vi "Main.vi"(11 "Module Admin":refnum<class "Delacor_lib_QMH_Module Admin.lvclass">) -> ()   [LabVIEW 2019, in "ContextHelp.lvlib"]
doc: "This template is based off of the Queued Message Handler design pattern and the Queued Message Handler project template that ships with LabVIEW.\n\nThe main difference is that the queue is private to this module and communication between modules is performed via Broadcast and Request events.\n\nRequest events are wrapped in public API methods and are handled in the Event Handling Loop (EHL) of this VI. Any module can register for Broadcast events sent by this module. The EHL generates messages based on user interface actions.\n\nThe Message Handling Loop (MHL) processes messages generated by the EHL, or by other messages. The messages are string values, so new messages can be added easily to the Message Cases case structure in the MHL. Each message cluster can also provide an optional value for Message Data, which is a variant that can be converted to whatever message-specific data is required.\n_____\nBased on DQMH Project Template 6.1.0.94.\n____\nPantherLAB Templates 1.0.0.5\nCopyright (c) 2022, PantherLAB\n\n<b>Note:</b> This VI was modified by the <b>Validate DQMH Module</b> tool to add a 'Panel Hidden' status updated broadcast to the Panel Close? event when External Launch = TRUE.\n\n<b>Note:</b> This VI was modified by the <b>Validate DQMH Module</b> tool to add a call to the Error Reported VI at the end of the 'Exit' MHL frame."
uses:
  ContextHelp.lvlib
  <vilib>/Delacor/Delacor QMH/Libraries/Module Admin_class/Delacor_lib_QMH_Module Admin.lvclass
  Module Data--cluster.ctl
  <vilib>/Delacor/Delacor QMH/Libraries/Message Queue_class/Delacor_lib_QMH_Message Queue.lvclass/Delacor_lib_QMH_Message Queue.ctl
  <vilib>/Utility/miscctls.llb/LVTextColorsTypeDef.ctl
  Stop Argument--cluster.ctl
  <vilib>/Delacor/Delacor QMH/Libraries/Module Admin_class/Delacor_lib_QMH_Module Admin.lvclass/Delacor_lib_QMH_Module Admin.ctl
  Draw Panel Into Subpanel Argument--cluster.ctl
  Remove Panel from Subpanel Argument--cluster.ctl
  <vilib>/Delacor/Delacor QMH/Libraries/Message Queue_class/Delacor_lib_QMH_Enqueue Message (Single).vi
  <vilib>/Delacor/Delacor QMH/Libraries/Module Admin_class/Delacor_lib_QMH_Get External Launch.vi
  <vilib>/Utility/error.llb/Error Cluster From Error Code.vi
  <vilib>/ErrorRing/Error Ring.xnode
  <vilib>/Delacor/Delacor QMH/Libraries/Message Queue_class/Delacor_lib_QMH_Message Queue.lvclass
  Panther Dashboard/Panther Dashboard.lvlib
panel:
  out "Status":string
  out "error out":errorcluster
  out "DQMH Version":string
  in  "Edit Project Description":bool caption="Project Description"
  in  "Project Description":string
  in  "Edit Module Description":bool caption="Module Description"
  in  "Module Description":string
  in  "Edit VI":bool caption="Event Description"
  out "Event Connector Pane":picture
  in  "Event Description":string
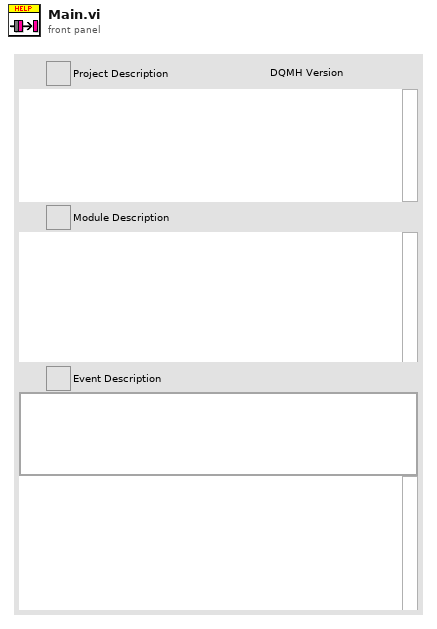
[diagram p1: front panel]
types:
  T1 = typedef "Panther Dashboard.lvlib/Broadcast Events--cluster.ctl" = cluster{"Module Did Init":refnum<user-event>, "Status Updated":refnum<user-event>, "Error Reported":refnum<user-event>, "Module Did Stop":refnum<user-event>, "Update Module Execution Status":refnum<user-event>, "References Updated":refnum<user-event>, "Projects Updated":refnum<user-event>, "Targets Updated":refnum<user-event>, "Progress updated":refnum<user-event>, "Scale Updated":refnum<user-event>, "Connector Pane Updated":refnum<user-event>, "Documentation Updated":refnum<user-event>, "Module Type Updated":refnum<user-event>, "Theme Updated":refnum<user-event>, "Project Description Updated":refnum<user-event>}
  T2 = typedef "ContextHelp.lvlib/Request Events--cluster.ctl" = cluster{"Stop Module":refnum<user-event>, "Show Panel":refnum<user-event>, "Hide Panel":refnum<user-event>, "Get Module Execution Status":refnum<user-event>, "Show Diagram":refnum<user-event>, "Draw Panel Into Subpanel":refnum<user-event>, "Remove Panel from Subpanel":refnum<user-event>, "Refresh Panther Dashboard Broadcasts":refnum<user-event>}
  T3 = typedef "ContextHelp.lvlib/Module Data--cluster.ctl" = cluster{"Status":string, "SubPanel":refnum<vi>, "Panel Status":bool}
  T4 = enum8{"Enabled", "Disabled", "Disabled and Grayed Out"}
  T5 = typedef "LVTextColorsTypeDef.ctl" = cluster{"Text Color":u32, "Background Color":u32}
  T6 = enum32{"invalid lock state", "Not Locked", "Locked (No Password)", "Password-protected"}
  T7 = typedef "ContextHelp.lvlib/Stop Argument--cluster.ctl" = cluster{"Origin":string, "Exit via Stop Module Req?":bool, "Wait for Module to stop?":bool}
  T8 = typedef "ContextHelp.lvlib/Draw Panel Into Subpanel Argument--cluster.ctl" = cluster{"Sub Panel":refnum<vi>}
  T9 = typedef "ContextHelp.lvlib/Remove Panel from Subpanel Argument--cluster.ctl" = cluster{"Boolean":bool}
  T10 = enum32{"Invalid", "Standard", "Closed", "Hidden", "Minimized", "Maximized"}
  T11 = typedef "Panther Dashboard.lvlib/Documentation--cluster.ctl" = cluster{"Module Description":string, "Event Description":string}
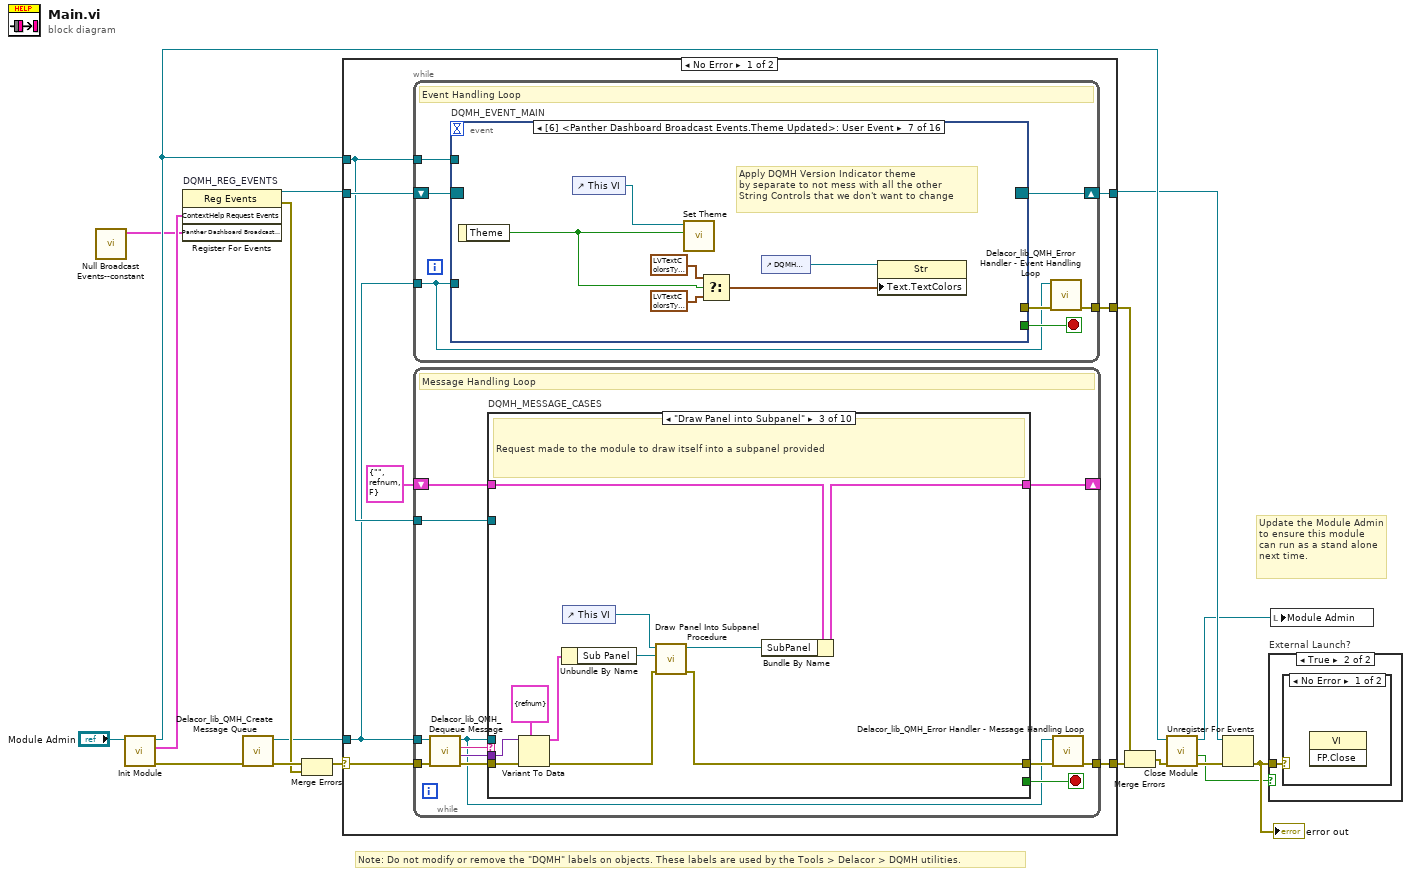
[diagram p0: block diagram]
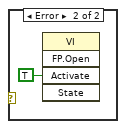
[diagram p3: hidden frame]
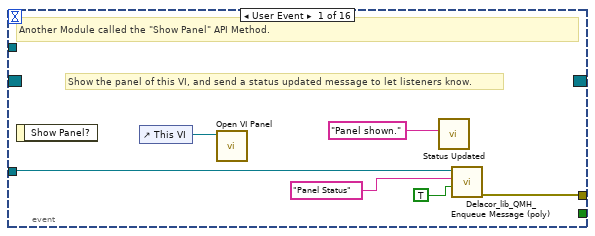
[diagram p4: hidden frame]
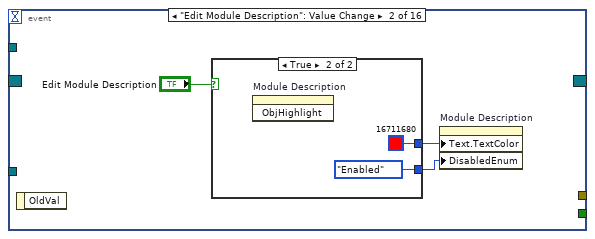
[diagram p5: hidden frame]
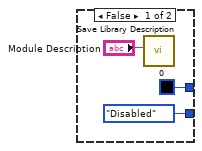
[diagram p6: hidden frame]
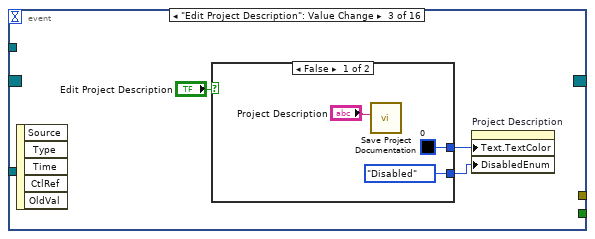
[diagram p7: hidden frame]
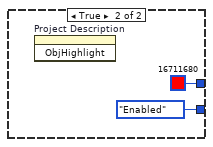
[diagram p8: hidden frame]
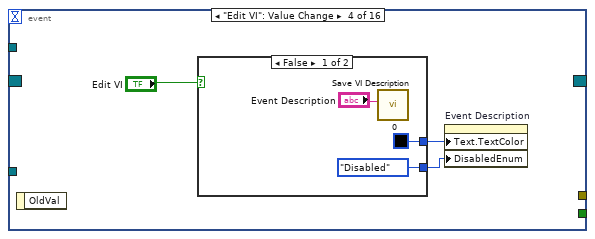
[diagram p9: hidden frame]
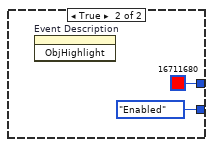
[diagram p10: hidden frame]
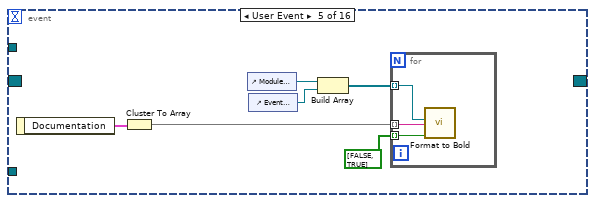
[diagram p11: hidden frame]
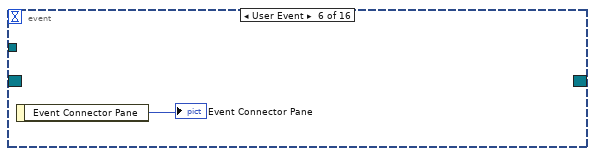
[diagram p12: hidden frame]
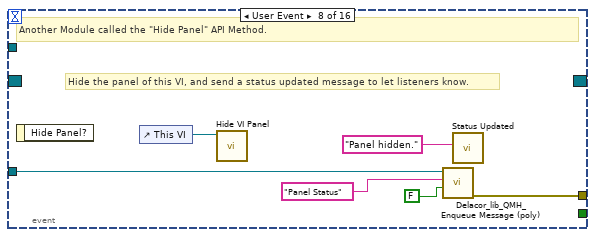
[diagram p13: hidden frame]
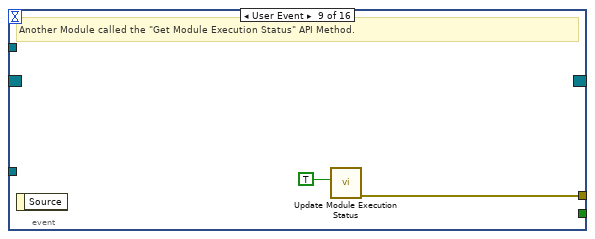
[diagram p14: hidden frame]
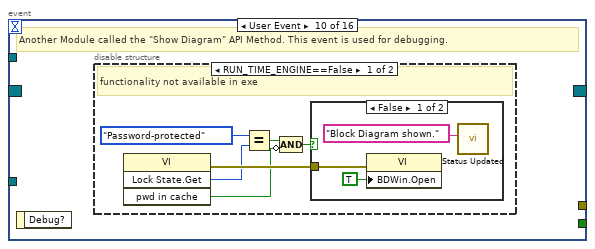
[diagram p15: hidden frame]
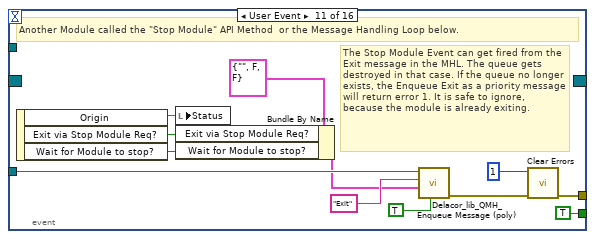
[diagram p18: hidden frame]
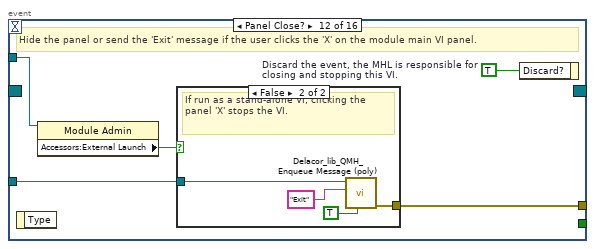
[diagram p19: hidden frame]
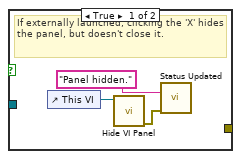
[diagram p20: hidden frame]
diagram:
  # "Note: Do not modify or remove the \"DQMH\" labels on objects. These labels are used by the Tools > Delacor > DQMH utilities."
  # "Update the Module Admin to ensure this module can run as a stand alone next time."
  n1 = call "Null Broadcast Events--constant.vi"() -> ("Panther Dashboard Broadcast Events"=w1:T1)  [unwired: 11 in]
  n2 = call "Init Module.vi"("Singleton Module Admin in"="Module Admin") -> ("error out"=w17:errorcluster, "ContextHelp Request Events"=w2:T2, "Singleton Module Admin out"=w9:refnum<class "Delacor_lib_QMH_Module Admin.lvclass">)  [unwired: 8 in]
  n3 = register-events "DQMH_REG_EVENTS"(w2, w1) -> (reference out=w7:refnum<event-registration>, error out=w10:errorcluster)  [unwired: 2 in]
  n4 = call <vilib>:"Delacor_lib_QMH_Create Message Queue.vi"("error in"=w17) -> ("error out"=w12:errorcluster, "Message Queue"=w6:refnum<class "Delacor_lib_QMH_Message Queue.lvclass">)  [unwired: 9 in]
  n5 = Merge Errors(w12, w10) -> (w11:errorcluster)
  n6 = case shown="No Error" w11 {
    selector: w11 -> [w24 w258]
    tunnel: [w26 w257] -> w18
    tunnel: [w23 w256] -> w8
    tunnel: w7 -> [w21 w256]
    tunnel: w6 -> [w19 w251]
    tunnel: [w25 _] -> w15
    tunnel: w9 -> [w20 w252]
    frame No Error {
      n7 = while {
        tunnel: w19 -> [w27]
        shift-right: [w30] -> w23
        shift-left: w21 -> [w31]
        tunnel: [w32] -> w25
        tunnel: w20 -> [w28]
        stop <- w29 stop-if-true
        # "Event Handling Loop"
        n8 = event "DQMH_EVENT_MAIN" shown="[6] <Panther Dashboard Broadcast Events.Theme Updated>: User Event" {
          selector: w31 -> [_ _ _ _ _ _ _ _ _ _ _ _ _ _ w135 _]
          dyn-events: [_ _ _ _ _ _ _ _ _ _ _ _ _ _ w134 _] -> w30
          timeout: _ -> [_ _ _ _ _ _ _ _ _ _ _ _ _ _ _ _]
          tunnel: [_ _ _ _ _ _ _ _ _ _ TRUE ("Discard?") _ _ _ _ _] -> w29
          tunnel: w27 -> [w36 _ _ _ _ _ _ w80 _ _ w104 w111 w125 w131 _ _]
          tunnel: [w39 _ _ _ _ _ _ w85 w87 _ w107 w113 w126 w132 _ _] -> w33
          tunnel: w28 -> [_ _ _ _ _ _ _ _ _ _ _ w110 _ _ _ _]
          event User Event {
            # "Show the panel of this VI, and send a status updated message to let listeners know."
            # "Another Module called the \"Show Panel\" API Method."
            n9 = event-data() -> ()  [unwired: 1 in, 1 out]
            n10 = control-ref of="This VI"() -> (w38:refnum<vi>)
            n11 = call "Open VI Panel.vi"("VI"=w38) -> ()  [unwired: 10 in, 1 out]
            n12 = call "Status Updated.vi"("Status"="Panel shown." ("format string")) -> ()  [unwired: 10 in, 1 out]
            n13 = call-poly <vilib>:"Delacor_lib_QMH_Enqueue Message (poly).vi"("Message Data"=TRUE, "Message"="Panel Status" ("format string"), "Message Queue in"=w36) -> ("error out"=w39:errorcluster)  [unwired: 7 in, 1 out]
          }
          event "Edit Module Description": Value Change {
            n14 = event-data() -> ()  [unwired: 1 in, 1 out]
            n15 = case shown="True" "Edit Module Description" {
              tunnel: [u32 0 u32 16711680] -> w41
              tunnel: [T4."Disabled" ("Disabled") T4."Enabled" ("Disabled")] -> w42
              frame False {
                n16 = call "Save Library Description.vi"("Library Description"="Module Description") -> ()  [unwired: 10 in, 1 out]
              }
              frame True {
                n17 = invoke on="Module Description" class="Str" method="ObjHighlight"() -> ()  [unwired: 3 in, 3 out]
              }
            }
            n18 = property on="Module Description" class="Str"("Text.TextColor"=w41, "DisabledEnum"=w42) -> ()  [unwired: 2 in, 2 out]
          }
          event "Edit Project Description": Value Change {
            n19 = event-data() -> ()  [unwired: 1 in, 5 out]
            n20 = case shown="False" "Edit Project Description" {
              tunnel: [u32 0 u32 16711680] -> w49
              tunnel: [T4."Disabled" ("Disabled") T4."Enabled" ("Disabled")] -> w50
              frame False {
                n21 = call "Save Project Documentation.vi"("Project Description"="Project Description") -> ()  [unwired: 10 in, 1 out]
              }
              frame True {
                n22 = invoke on="Project Description" class="Str" method="ObjHighlight"() -> ()  [unwired: 3 in, 3 out]
              }
            }
            n23 = property on="Project Description" class="Str"("Text.TextColor"=w49, "DisabledEnum"=w50) -> ()  [unwired: 2 in, 2 out]
          }
          event "Edit VI": Value Change {
            n24 = event-data() -> ()  [unwired: 1 in, 1 out]
            n25 = case shown="False" "Edit VI" {
              tunnel: [u32 0 u32 16711680] -> w57
              tunnel: [T4."Disabled" ("Disabled") T4."Enabled" ("Disabled")] -> w58
              frame False {
                n26 = call "Save VI Description.vi"("VI Description"="Event Description") -> ()  [unwired: 10 in, 1 out]
              }
              frame True {
                n27 = invoke on="Event Description" class="Str" method="ObjHighlight"() -> ()  [unwired: 3 in, 3 out]
              }
            }
            n28 = property on="Event Description" class="Str"("Text.TextColor"=w57, "DisabledEnum"=w58) -> ()  [unwired: 2 in, 2 out]
          }
          event User Event {
            n29 = event-data() -> ("Documentation"=w69:T11)  [unwired: 1 in]
            n30 = Cluster To Array(cluster=w69) -> (array=w67:string[])
            n31 = control-ref of="Module Description"() -> (w65:refnum<vi>)
            n32 = control-ref of="Event Description"() -> (w64:refnum<vi>)
            n33 = Build Array(w65, w64) -> (w66:refnum<vi>[])
            n34 = for {
              tunnel: bool[] [FALSE, TRUE] ("Adjust Height?") -> [w72] mode=indexing
              tunnel: w67 -> [w71] mode=indexing
              tunnel: w66 -> [w70] mode=indexing
              n35 = call "Format to Bold.vi"("Adjust Height?"=w72, "String Value"=w71, "String Ref"=w70) -> ()  [unwired: 9 in]
            }
          }
          event User Event {
            n36 = event-data() -> ("Event Connector Pane"=→"Event Connector Pane":picture)  [unwired: 1 in]
          }
          event User Event {
            # "Apply DQMH Version Indicator theme\nby separate to not mess with all the other\nString Controls that we don't want to change"
            n37 = event-data() -> ("Theme"=w76:bool)  [unwired: 1 in]
            n38 = control-ref of="This VI"() -> (w79:refnum<vi>)
            n39 = call "Set Theme.vi"("Dark?"=w76, "VI in"=w79) -> ()  [unwired: 10 in]
            n40 = Select(t=T5 {"Text Color"=16448250, "Background Color"=16777216} ("Label.Text Colors"), s=w76, f=T5 {"Text Color"=0, "Background Color"=16777216} ("Label.Text Colors")) -> (s? t:f=w74:T5)
            n41 = control-ref of="DQMH Version"() -> (w75:refnum<vi>)
            n42 = property class="Str"(reference=w75, "Text.TextColors"=w74) -> ()  [unwired: 1 in, 2 out]
          }
          event User Event {
            # "Hide the panel of this VI, and send a status updated message to let listeners know."
            # "Another Module called the \"Hide Panel\" API Method."
            n43 = event-data() -> ()  [unwired: 1 in, 1 out]
            n44 = control-ref of="This VI"() -> (w84:refnum<vi>)
            n45 = call "Hide VI Panel.vi"("VI"=w84) -> ()  [unwired: 10 in, 1 out]
            n46 = call-poly <vilib>:"Delacor_lib_QMH_Enqueue Message (poly).vi"("Message Data"=FALSE, "Message"="Panel Status" ("format string"), "Message Queue in"=w80) -> ("error out"=w85:errorcluster)  [unwired: 7 in, 1 out]
            n47 = call "Status Updated.vi"("Status"="Panel hidden." ("format string")) -> ()  [unwired: 10 in, 1 out]
          }
          event User Event {
            # "Another Module called the \"Get Module Execution Status\" API Method."
            n48 = event-data() -> ()  [unwired: 1 in, 1 out]
            n49 = call "Update Module Execution Status.vi"("Running?"=TRUE) -> ("error out"=w87:errorcluster)  [unwired: 10 in]
          }
          event User Event {
            # "Another Module called the \"Show Diagram\" API Method. This event is used for debugging."
            n50 = event-data() -> ()  [unwired: 1 in, 1 out]
            n51 = disable-structure shown="RUN_TIME_ENGINE==False" {
              frame condition #0 (active) {
                # "functionality not available in exe"
                n52 = invoke class="VI" method="Lock State.Get"() -> (error out=w93:errorcluster, "Get Lock State"=w92:T6, "pwd in cache"=w89:bool)  [unwired: 4 in, 1 out]
                n53 = Equal?(x=T6."Password-protected", y=w92) -> (x = y?=w90:bool)
                n54 = Compound Arithmetic op=AND(w90, invert w89) -> (w88:bool)
                n55 = case shown="False" w88 {
                  tunnel: w93 -> [w96 _]
                  frame False {
                    n56 = property class="VI"(error in=w96, "BDWin.Open"=TRUE ("Block Diagram Window:Open")) -> ()  [unwired: 1 in, 2 out]
                    n57 = call "Status Updated.vi"("Status"="Block Diagram shown." ("format string")) -> ()  [unwired: 10 in, 1 out]
                  }
                  frame True {
                    # "Password-protected VI, and the password is not in the cache. Do not show the diagram."
                  }
                }
              }
              frame condition #1 {
              }
            }
          }
          event User Event {
            # "The Stop Module Event can get fired from the Exit message in the MHL. The queue gets destroyed in that case. If the queue no longer exists, the Enqueue Exit as a priority message will return error 1. It is safe to ignore, because the module is already exiting."
            # "Another Module called the \"Stop Module\" API Method  or the Message Handling Loop below."
            n58 = event-data() -> ("Origin"=w103:string, "Exit via Stop Module Req?"=w99:bool, "Wait for Module to stop?"=w98:bool)  [unwired: 1 in]
            n59 = local write "Status"(w103) -> ()
            n60 = Bundle By Name(cluster=T7 {"Origin"="", "Exit via Stop Module Req?"=FALSE, "Wait for Module to stop?"=FALSE} ("Stop Argument"), "Exit via Stop Module Req?"=w99, "Wait for Module to stop?"=w98) -> (w97:T7)
            n61 = call-poly <vilib>:"Delacor_lib_QMH_Enqueue Message (poly).vi"("Priority Message? (F)"=TRUE, "Message Data"=w97, "Message"="Exit", "Message Queue in"=w104) -> ("error out"=w108:errorcluster)  [unwired: 6 in, 1 out]
            n62 = call <vilib>:"Clear Errors.vi"("error in (no error)"=w108, "specific error code to clear (0: all)"=1) -> ("error out"=w107:errorcluster)  [unwired: 4 in, 1 out]
          }
          event Panel Close? {
            w112 = TRUE  # Discard the event, the MHL is responsible for closing and stopping this VI.
            # "Hide the panel or send the 'Exit' message if the user clicks the 'X' on the module main VI panel."
            n63 = event-data() -> ()  [unwired: 1 in, 1 out]
            n64 = property class="Module Admin"(reference=w110) -> ("Accessors:External Launch"=w109:bool)  [unwired: 1 in, 2 out]
            n65 = case shown="False" w109 {
              tunnel: w111 -> [_ w119]
              tunnel: [_ w120] -> w113
              frame True {
                # "If externally launched, clicking the 'X' hides the panel, but doesn't close it."
                n66 = control-ref of="This VI"() -> (w116:refnum<vi>)
                n67 = call "Hide VI Panel.vi"("VI"=w116) -> ("error out"=w114:errorcluster)  [unwired: 10 in]
                n68 = call "Status Updated.vi"("error in (no error)"=w114, "Status"="Panel hidden.") -> ()  [unwired: 9 in, 1 out]
              }
              frame False {
                # "If run as a stand-alone VI, clicking the panel 'X' stops the VI."
                n69 = call-poly <vilib>:"Delacor_lib_QMH_Enqueue Message (poly).vi"("Priority Message? (F)"=TRUE, "Message"="Exit", "Message Queue in"=w119) -> ("error out"=w120:errorcluster)  [unwired: 7 in, 1 out]
              }
            }
            n70 = event-data("Discard?"=w112) -> ()  [unwired: 1 in, 1 out]
          }
          event User Event {
            # "Another Module called the \"Draw your Panel into Subpanel\" API Method."
            n71 = event-data() -> ("Sub Panel"=w121:refnum<vi>)  [unwired: 1 in]
            n72 = Bundle(cluster=T8 {"Sub Panel"=refnum} ("Draw your Panel into Subpanel Argument"), "Sub Panel"=w121) -> (w122:T8)
            n73 = call-poly <vilib>:"Delacor_lib_QMH_Enqueue Message (poly).vi"("Message Data"=w122, "Message"="Draw Panel into Subpanel", "Message Queue in"=w125) -> ("error out"=w126:errorcluster)  [unwired: 7 in, 1 out]
          }
          event User Event {
            # "Another Module called the \"Remove Panel from Subpanel\" API Method."
            n74 = event-data() -> ("Boolean"=w127:bool)  [unwired: 1 in]
            n75 = Bundle(cluster=T9 {"Boolean"=FALSE} ("Remove Panel from Subpanel Argument"), "Boolean"=w127) -> (w128:T9)
            n76 = call-poly <vilib>:"Delacor_lib_QMH_Enqueue Message (poly).vi"("Message Data"=w128, "Message"="Remove Panel from Subpanel", "Message Queue in"=w131) -> ("error out"=w132:errorcluster)  [unwired: 7 in, 1 out]
          }
          event User Event {
            # "Another Module called the \"Refresh Panther Dashboard Broadcasts\" API Method."
            n77 = event-data() -> ()  [unwired: 1 in, 1 out]
            n78 = call "Obtain Broadcast Events for Registration.vi"() -> ("Panther Dashboard Broadcast Events"=w133:T1)  [unwired: 9 in, 2 out]
            n79 = register-events "Refresh Panther Broadcasts"(reference=w135, w133) -> (reference out=w134:refnum<event-registration>)  [unwired: 2 in, 1 out]
          }
          event User Event {
            n80 = event-data() -> ("Project Description"=w136:string)  [unwired: 1 in]
            n81 = local write "Project Description"(w136) -> ()
          }
        }
        n82 = call-dynamic "Delacor_lib_QMH_Error Handler - Event Handling Loop.vi"("error in"=w33, "Message Queue in"=w27) -> ("dup error in"=w32:errorcluster)  [unwired: 8 in, 1 out]
      }
      n83 = while {
        tunnel: w19 -> [w139]
        shift-right: [w143] -> _
        shift-left: T3 {"Status"="", "SubPanel"=refnum, "Panel Status"=FALSE} ("Data Cluster") -> [w144]
        tunnel: w24 -> [w147]
        tunnel: [w145] -> w26
        tunnel: w20 -> [w137]
        stop <- w142 stop-if-true
        # "Message Handling Loop"
        n84 = call-dynamic "Delacor_lib_QMH_Dequeue Message.vi"("error in"=w147, "Message Queue in"=w139) -> ("error out"=w146:errorcluster, "Message Data"=w140:variant, "Message"=w141:string, "Message Queue out"=w138:refnum<class "Delacor_lib_QMH_Message Queue.lvclass">)  [unwired: 6 in]
        n85 = case "DQMH_MESSAGE_CASES" shown="\"Draw Panel into Subpanel\"" w141 {
          selector: w141 -> [_ _ _ _ _ _ _ _ _ w238]
          tunnel: w138 -> [_ _ _ _ _ _ _ w207 w230 _]
          tunnel: w146 -> [w166 w170 w181 w190 w199 w202 w204 w214 w236 w240]
          tunnel: [w164 w170 w179 w189 w198 w201 w204 w210 w233 w241] -> w148
          tunnel: w144 -> [w156 w169 w178 w185 w197 w200 w203 w209 w222 w239]
          tunnel: [w155 w169 w172 w185 w194 w200 w203 w209 w222 w239] -> w143
          tunnel: [_ _ _ _ _ _ _ _ w229 _] -> w142
          tunnel: w140 -> [_ _ w177 w187 w196 _ _ w208 w228 _]
          tunnel: w137 -> [w157 _ _ _ _ _ _ w206 w223 _]
          frame "Initialize" {
            w151 = "Initial Message" ("Initial Message")
            # "Initialize - Any operation that needs to be done before the module can receive messages. Synchronize Caller Events.vi will inform Start Module.vi that the module has launched and is ready to receive messages. Module Did Init.vi will broadcast that the module initialized."
            n86 = call "Synchronize Caller Events.vi"("error in (no error)"=w166, "Singleton Module Admin in"=w157) -> ("error out"=w165:errorcluster, "Singleton Module Admin out"=w152:refnum<class "Delacor_lib_QMH_Module Admin.lvclass">)  [unwired: 8 in]
            n87 = property class="Module Admin"(reference=w152) -> ("Accessors:External Launch"=w161:bool)  [unwired: 1 in, 2 out]
            n88 = call <vilib>:"DQMH_DQMH Version Information--constant.vi"() -> ("DQMH Version"=→"DQMH Version":string)  [unwired: 11 in]
            n89 = Select(t=T10."Hidden" ("State"), s=w161, f=T10."Standard" ("State")) -> (s? t:f=w158:T10)
            n90 = property class="VI"("Front Panel.Title"="DQMH Context Help" ("Front Panel Window:Title")) -> (reference out=w163:refnum<vi>, error out=w168:errorcluster)  [unwired: 2 in]
            n91 = call "Module Name--constant.vi"() -> ("Module Name"=w153:string)  [unwired: 11 in]
            n92 = invoke class="VI" method="FP.Open"(reference=w163, error in=w168, "State"=w158) -> (reference out=w162:refnum<vi>, error out=w167:errorcluster)  [unwired: 2 in, 3 out]
            n93 = call "Module Did Init.vi"("error in (no error)"=w165, "Initialized?"=TRUE, "Origin"=w153) -> ("error out"=w164:errorcluster)  [unwired: 8 in]
            n94 = Bundle By Name(cluster=w156, "Status"=w151) -> (w155:T3)
            n95 = invoke class="VI" method="FP.Center"(reference=w162, error in=w167) -> ()  [unwired: 1 in, 3 out]
            "Status" <- w151
          }
          frame "---Module Specific---" {
            # "Separator -- The following cases handle messages specific to this Module."
          }
          frame "Draw Panel into Subpanel" {
            # "Request made to the module to draw itself into a subpanel provided"
            n96 = Variant To Data(error in=w181, type=T8 {"Sub Panel"=refnum} ("Draw your Panel into Subpanel Argument"), Variant=w177) -> (data=w175:T8, error out=w180:errorcluster)
            n97 = Unbundle By Name(w175) -> ("Sub Panel"=w173:refnum<vi>)
            n98 = control-ref of="This VI"() -> (w174:refnum<vi>)
            n99 = call "Draw Panel Into Subpanel Procedure.vi"("error in"=w180, "SubPanel in"=w173, "This VI"=w174) -> ("error out"=w179:errorcluster, "SubPanel out"=w171:refnum<vi>)  [unwired: 7 in]
            n100 = Bundle By Name(cluster=w178, "SubPanel"=w171) -> (w172:T3)
          }
          frame "Remove Panel from Subpanel" {
            # "Request to the module to remove itself from the subpanel"
            n101 = Variant To Data(error in=w190, type=T9 {"Boolean"=FALSE} ("Remove Panel from Subpanel Argument"), Variant=w187) -> (error out=w189:errorcluster)  [unwired: 1 out]
            n102 = Unbundle By Name(w185) -> ("Panel Status"=w183:bool, "SubPanel"=w184:refnum<vi>)
            n103 = invoke class="SubPnl" method="Remove VI"(reference=w184) -> (error out=w188:errorcluster)  [unwired: 2 in, 2 out]
            n104 = control-ref of="This VI"() -> (w182:refnum<vi>)
            n105 = case shown="False" w183 {
              tunnel: w188 -> [_ _]
              tunnel: w182 -> [w191 w192]
              frame False {
                # "Hiden"
                n106 = call "Hide VI Panel.vi"("VI"=w191) -> ()  [unwired: 10 in, 1 out]
              }
              frame True {
                # "Visible"
                n107 = call "Open VI Panel.vi"("VI"=w192) -> ()  [unwired: 10 in, 1 out]
              }
            }
          }
          frame "Panel Status" {
            n108 = Variant To Data(error in=w199, type=TRUE, Variant=w196) -> (data=w193:bool, error out=w198:errorcluster)
            n109 = Bundle By Name(cluster=w197, "Panel Status"=w193) -> (w194:T3)
          }
          frame "---Copy This Frame---" {
            # "Duplicate this frame when creating new messages.  Change this comment in the duplicated frame to describe this message."
            n110 = Merge Errors(w202) -> (w201:errorcluster)
          }
          frame "---Exit and Error Handling---" {
            # "Separator - The following cases handle errors and exit messages."
          }
          frame "Error" {
            # "Error - Check the error message data and respond accordingly. This message is sent by the \"Error Handler\" VIs at the end of each loop in this application."
            n111 = property class="Module Admin"(reference=w206) -> ("Accessors:External Launch"=w205:bool)  [unwired: 1 in, 2 out]
            n112 = Variant To Data(error in=w214, type=errorcluster {"status"=FALSE, "code"=0, "source"=""} ("error constant"), Variant=w208) -> (data=w215:errorcluster, error out=w212:errorcluster)
            n113 = call "Error Reported.vi"("Error"=w215) -> ()  [unwired: 10 in, 1 out]
            n114 = case shown="False" w205 {
              tunnel: [w220 _] -> w211
              tunnel: w207 -> [w218 _]
              tunnel: w215 -> [w219 _]
              frame False {
                # "If the module is running standalone, then pop up an error dialog and call the \"Exit\" message."
                n115 = call <vilib>:"Simple Error Handler.vi"("error in (no error)"=w219) -> ()  [unwired: 4 in, 5 out]
                n116 = call-poly <vilib>:"Delacor_lib_QMH_Enqueue Message (poly).vi"("Priority Message? (F)"=TRUE, "Message"="Exit", "Message Queue in"=w218) -> ("error out"=w220:errorcluster)  [unwired: 7 in, 1 out]
              }
              frame True {
                # "If the module was launched externally, calling the Error Reported broadcast VI is the only action performed by the \"Error\" message. The module's caller can then process the error appropriately."
              }
            }
            n117 = Merge Errors(w212, w211) -> (w210:errorcluster)
            n118 = local write "error out"(w210) -> ()
          }
          frame "Exit" {
            w227 = 91  # 91: not all Exit messages will have an argument
            w229 = TRUE  # Stop the VI
            # "Release the message queue reference"
            # "Exit - Exit the application."
            n119 = Variant To Data(error in=w236, type=T7 {"Origin"="", "Exit via Stop Module Req?"=FALSE, "Wait for Module to stop?"=FALSE} ("Stop Argument"), Variant=w228) -> (data=w225:T7, error out=w232:errorcluster)
            n120 = call <vilib>:"Clear Errors.vi"("error in (no error)"=w232, "specific error code to clear (0: all)"=w227) -> ("error out"=w235:errorcluster)  [unwired: 4 in, 1 out]
            n121 = Unbundle By Name(w222) -> ("SubPanel"=w221:refnum<vi>)
            n122 = control-ref of="This VI"() -> (w224:refnum<vi>)
            n123 = invoke class="SubPnl" method="Remove VI"(reference=w221) -> ()  [unwired: 2 in, 3 out]
            n124 = call-dynamic "Delacor_lib_QMH_Release Message Queue.vi"("error in"=w235, "Message Queue"=w230) -> ("error out"=w234:errorcluster)  [unwired: 9 in]
            n125 = call "Handle Exit.vi"("Stop Argument"=w225, "Admin in"=w223, "VI reference"=w224) -> ("error out"=w231:errorcluster)  [unwired: 7 in, 1 out]
            n126 = Merge Errors(w234, w231) -> (w233:errorcluster)
            n127 = call "Error Reported.vi"("Error"=w233) -> ()  [unwired: 10 in, 1 out]
          }
          frame Default {
            # "'Default' case only runs if there is a message that isn't defined in any of the other cases.  Output a programming error."
            n128 = call "Module Name--constant.vi"() -> ("Module Name"=w237:string)  [unwired: 11 in]
            n129 = xnode "Error Ring"("parameter 0"=w238, "parameter 1"=w237) -> ("error out"=w242:errorcluster)
            n130 = Merge Errors(w240, w242) -> (w241:errorcluster)
          }
        }
        n131 = call-dynamic "Delacor_lib_QMH_Error Handler - Message Handling Loop.vi"("error in"=w148, "Message Queue in"=w138) -> ("dup error in"=w145:errorcluster)  [unwired: 8 in, 1 out]
      }
    }
    frame Error {
      # "Synchronize Caller Events.vi will inform Start Module.vi that the module has launched and will let the code calling Start Module.vi register for broadcasts and would permit the caller receive the broadcast that an error occurred at launch time."
      n132 = call-dynamic "Delacor_lib_QMH_Release Message Queue.vi"("error in"=w258, "Message Queue"=w251) -> ("error out"=w257:errorcluster)  [unwired: 9 in]
      n133 = call "Synchronize Caller Events.vi"("Singleton Module Admin in"=w252) -> ("error out"=w259:errorcluster)  [unwired: 9 in, 1 out]
      n134 = call "Module Name--constant.vi"() -> ("Module Name"=w255:string)  [unwired: 11 in]
      n135 = Format Into String(format string="An error occurred during initialization. %s is no longer running.", w255) -> (resulting string=w253:string)  [unwired: 2 in, 1 out]
      n136 = Merge Errors(w257, w259) -> (w260:errorcluster)
      n137 = call "Error Reported.vi"("Additional Information"=w253, "Error"=w260) -> ()  [unwired: 9 in, 1 out]
    }
  }
  n138 = Merge Errors(w15, w18) -> (w14:errorcluster)
  n139 = call "Close Module.vi"("error in (no error)"=w14, "Module Admin in"=w9) -> ("error out"=w16:errorcluster, "External Launch"=w3:bool, "Module Admin out"=w4:refnum<class "Delacor_lib_QMH_Module Admin.lvclass">)  [unwired: 7 in]
  n140 = Unregister For Events(event registration refnum=w8, error in=w16) -> (error out=w13:errorcluster)
  "error out" <- w13
  n141 = case "External Launch?" shown="True" w3 {
    tunnel: w13 -> [_ w261]
    frame False {
    }
    frame True {
      n142 = case shown="No Error" w261 {
        frame No Error {
          n143 = invoke class="VI" method="FP.Close"() -> ()  [unwired: 3 in, 3 out]
        }
        frame Error {
          n144 = invoke class="VI" method="FP.Open"("Activate"=TRUE ("Activate?")) -> ()  [unwired: 4 in, 5 out]
        }
      }
    }
  }
  n145 = local write "Module Admin"(w4) -> ()
